vi "QCA - DUT Start Rx Dll.vi"(0 "Rx_Chan":i32, 7 "Receive Config":T2={"Frequency, MHz"=2412, "Data Rate"="1,0,0", "Packet Count"=0, "RX Mac Address"="10:11:11:11:11:01", "TX Mac Address"="10:11:11:11:11:01", "BS Mac Address"="10:11:11:11:11:01", "Packet Length"=1000, "Broadcast"=FALSE}, 11 "error in (no error)":errorcluster) -> (14 "Command Sent":string, 15 "error out":errorcluster)   [LabVIEW 2011]
uses:
  Controls/Data Rates.ctl
  Controls/Parameter.ctl
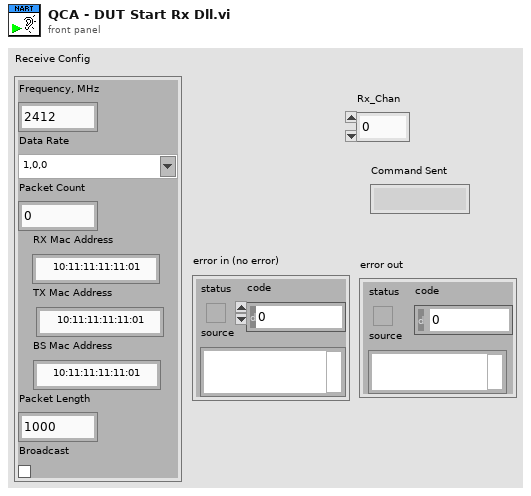
[diagram p1: front panel]
types:
  T1 = typedef "Data Rates.ctl" = string
  T2 = cluster{"Frequency, MHz":u32, "Data Rate":T1, "Packet Count":i32, "RX Mac Address":string, "TX Mac Address":string, "BS Mac Address":string, "Packet Length":u32, "Broadcast":bool}
  T3 = typedef "Parameter.ctl" = cluster{"Name":string, "Type":enum16{"decimal", "string", "float", "hex"}}
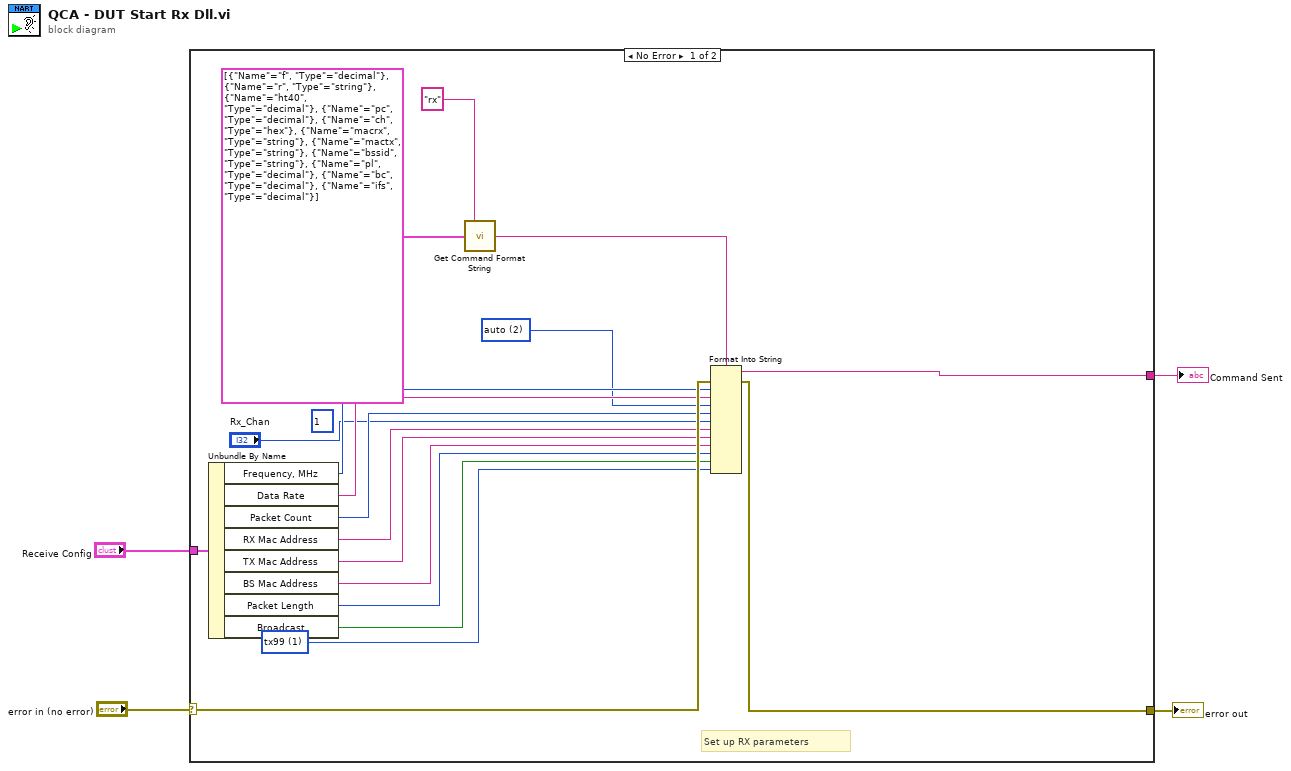
[diagram p0: block diagram]
diagram:
  n1 = case shown="No Error" "error in (no error)" {
    selector: "error in (no error)" -> [w20 w23]
    tunnel: [w7 w23] -> w3
    tunnel: "Receive Config" -> [w19 _]
    tunnel: [w6 _] -> w1
    frame No Error {
      w8 = i16 1 items=["Regular"=-1, "tx100"=0, "tx99"=1] ("Inter Frame Spacing")
      (unwired) 1 ("Chains")
      w9 = i16 2 items=["none"=0, "low"=-1, "high"=1, "auto"=2] ("input 3")
      # "Set up RX parameters"
      n2 = Unbundle By Name(w19) -> ("Frequency, MHz"=w17:u32, "Data Rate"=w10:T1, "Packet Count"=w16:i32, "RX Mac Address"=w15:string, "TX Mac Address"=w14:string, "BS Mac Address"=w12:string, "Packet Length"=w13:u32, "Broadcast"=w11:bool)
      n3 = call "Get Command Format String.vi"("Command"="rx", "Parameters"=T3[] [{"Name"="f", "Type"=enum."decimal"}, {"Name"="r", "Type"=enum."string"}, {"Name"="ht40", "Type"=enum."decimal"}, {"Name"="pc", "Type"=enum."decimal"}, {"Name"="ch", "Type"=enum."hex"}, {"Name"="macrx", "Type"=enum."string"}, {"Name"="mactx", "Type"=enum."string"}, {"Name"="bssid", "Type"=enum."string"}, {"Name"="pl", "Type"=enum."decimal"}, {"Name"="bc", "Type"=enum."decimal"}, {"Name"="ifs", "Type"=enum."decimal"}]) -> ("Command Format String"=w18:string)  [unwired: 13 in]
      n4 = Format Into String(format string=w18, error in=w20, w17, w10, w9, w16, "Rx_Chan", w15, w14, w12, w13, w11, w8) -> (resulting string=w6:string, error out=w7:errorcluster)  [unwired: 1 in]
    }
    frame Error {
    }
  }
  "error out" <- w3
  "Command Sent" <- w1
